vi "JumpToAnotherVI.vi"(8 "错误输入（无错误）":errorcluster, 10 "要关闭的VI":string, 11 "要打开的VI":string="Main.vi") -> (0 "错误输出":errorcluster)   [LabVIEW 2014]
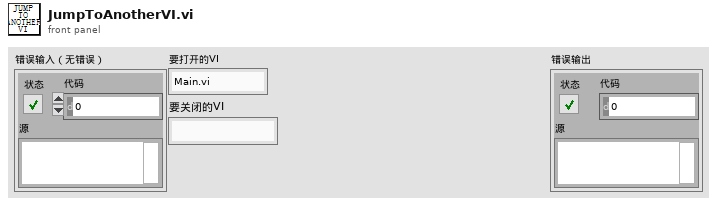
[diagram p1: front panel]
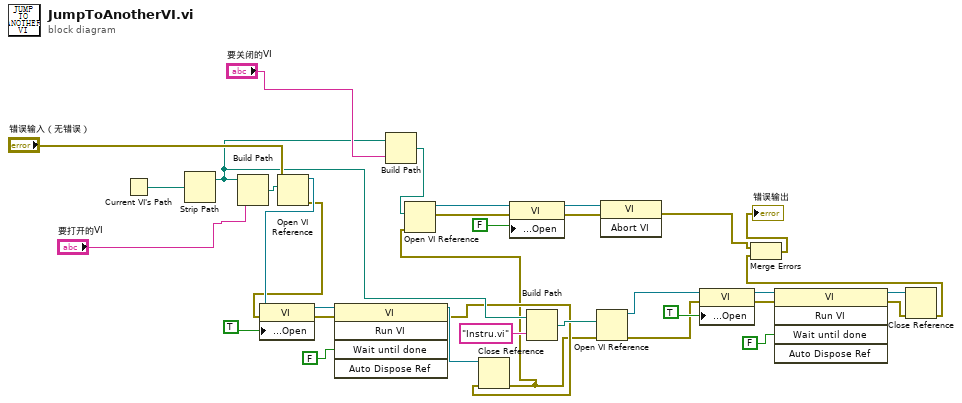
[diagram p0: block diagram]
diagram:
  n1 = Current VI's Path() -> (path=w22:path)
  n2 = Strip Path(path=w22) -> (stripped path=w17:path)  [unwired: 1 out]
  n3 = Build Path(base path=w17, name or relative path="要打开的VI") -> (appended path=w34:path)
  n4 = Open VI Reference(vi path=w34, error in (no error)="错误输入（无错误）") -> (vi reference=w29:refnum<vi>, error out=w28:errorcluster)  [unwired: 4 in]
  n5 = property on="Property Node" class="VI"(reference=w29, error in=w28, "Front Panel Window:Open"=TRUE) -> (reference out=w32:refnum<vi>, error out=w31:errorcluster)
  n6 = invoke class="VI" method="Run VI"(reference=w32, error in=w31, "Wait until done"=FALSE) -> (reference out=w14:refnum<vi>, error out=w13:errorcluster)  [unwired: 2 in, 3 out]
  n7 = Build Path(base path=w17, name or relative path="要关闭的VI") -> (appended path=w21:path)
  n8 = Close Reference(reference=w14, error in (no error)=w13) -> (error out=w4:errorcluster)
  n9 = Open VI Reference(vi path=w21, error in (no error)=w4) -> (vi reference=w27:refnum<vi>, error out=w25:errorcluster)  [unwired: 4 in]
  n10 = property on="Property Node" class="VI"(reference=w27, error in=w25, "Front Panel Window:Open"=FALSE) -> (reference out=w20:refnum<vi>, error out=w19:errorcluster)
  n11 = Build Path(base path=w17, name or relative path="Instru.vi" ("名称或相对路径")) -> (appended path=w15:path)
  n12 = Open VI Reference(vi path=w15, error in (no error)=w4) -> (vi reference=w9:refnum<vi>, error out=w8:errorcluster)  [unwired: 4 in]
  n13 = invoke class="VI" method="Abort VI"(reference=w20, error in=w19) -> (error out=w2:errorcluster)  [unwired: 1 in, 2 out]
  n14 = property on="Property Node" class="VI"(reference=w9, error in=w8, "Front Panel Window:Open"=TRUE) -> (reference out=w7:refnum<vi>, error out=w11:errorcluster)
  n15 = invoke class="VI" method="Run VI"(reference=w7, error in=w11, "Wait until done"=FALSE) -> (reference out=w6:refnum<vi>, error out=w5:errorcluster)  [unwired: 2 in, 3 out]
  n16 = Close Reference(reference=w6, error in (no error)=w5) -> (error out=w3:errorcluster)
  n17 = Merge Errors(w2, w3) -> (→"错误输出":errorcluster)
